vi "Set range.vi"(8 "error in":errorcluster, 10 "Range number {0 to 9}":u16 max=9, 11 "VISA resource name":refnum<visa-resource-name>) -> (0 "error out":errorcluster, 3 "VISA resource name out":refnum<visa-resource-name>)   [LabVIEW 2013, in "Datron D4xxx.lvlib"]
doc: "This VI sets instrument range."
uses:
  Datron D4xxx.lvlib
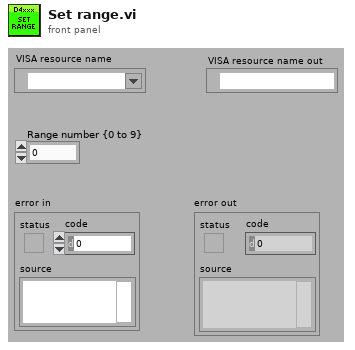
[diagram p1: front panel]
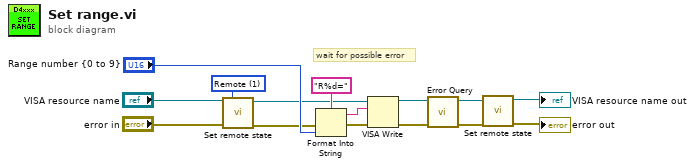
[diagram p0: block diagram]
diagram:
  w1 = u16 1 items=["Local", "Remote", "Default"] ("Remote state")
  # "wait for possible error"
  n1 = call "Set remote state.vi"("error in"="error in", "Remote state"=w1, "VISA resource name"="VISA resource name") -> ("error out"=w4:errorcluster, "VISA resource name out"=w2:refnum<visa-resource-name>)  [unwired: 7 in]
  n2 = Format Into String(format string="R%d=", error in=w4, "Range number {0 to 9}") -> (resulting string=w15:string, error out=w14:errorcluster)  [unwired: 1 in]
  n3 = VISA Write(VISA resource name=w2, write buffer=w15, error in (no error)=w14) -> (VISA resource name out=w6:refnum<visa-resource-name>, error out=w7:errorcluster)  [unwired: 1 out]
  n4 = call "Error Query.vi"("error in (no error)"=w7, "VISA resource name"=w6) -> ("error out"=w11:errorcluster, "VISA resource name out"=w9:refnum<visa-resource-name>)  [unwired: 6 in, 2 out]
  n5 = call "Set remote state.vi"("error in"=w11, "VISA resource name"=w9) -> ("error out"=→"error out":errorcluster, "VISA resource name out"=→"VISA resource name out":refnum<visa-resource-name>)  [unwired: 8 in]
